vi "FindUniqueName.vi"(10 "Max Length":i32, 11 "PathIn":path) -> (3 "UniquedPath":path)   [LabVIEW 2015]
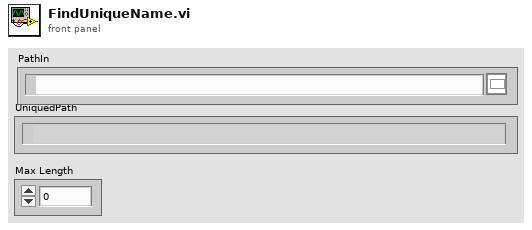
[diagram p1: front panel]
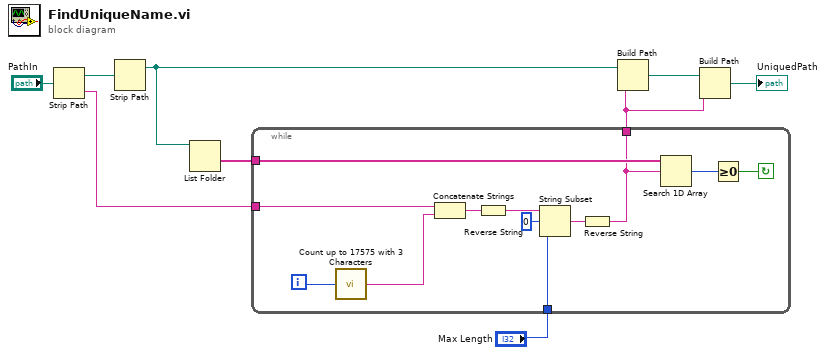
[diagram p0: block diagram]
diagram:
  n1 = Strip Path(path="PathIn") -> (stripped path=w3:path, name=w4:string)
  n2 = Strip Path(path=w3) -> (stripped path=w6:path)  [unwired: 1 out]
  n3 = List Folder(path=w6) -> (folder names=w5:string[])  [unwired: 1 in, 5 out]
  n4 = while {
    tunnel: w4 -> [w21]
    tunnel: "Max Length" -> [w20]
    tunnel: [w14] -> w7
    tunnel: w5 -> [w15]
    i -> [w11]
    stop <- w12 continue-if-true
    n5 = call "Count up to 17575 with 3 Characters.vi"("Numeric Control"=w11) -> ("string"=w10:string)
    n6 = Concatenate Strings(w21, w10) -> (w18:string)
    n7 = Reverse String(1:w18) -> (0:w19:string)
    n8 = String Subset(string=w19, offset (0)=0, length (rest)=w20) -> (substring=w17:string)
    n9 = Reverse String(1:w17) -> (0:w14:string)
    n10 = Search 1D Array(1D array=w15, element=w14) -> (index of element=w13:i32)  [unwired: 1 out]
    n11 = Greater Or Equal To 0?(x=w13) -> (x >= 0?=w12:bool)
  }
  n12 = Build Path(base path=w6, name or relative path=w7) -> (appended path=w8:path)
  n13 = Build Path(base path=w8, name or relative path=w7) -> (appended path=→"UniquedPath":path)
